vi "Calculate Friction Force.vi"(8 "error in":errorcluster, 10 "Mover Velocity in":refnum<class "PVector.lvclass">, 11 "Friction in":refnum<class "Friction.lvclass">) -> (0 "error out":errorcluster, 2 "Friction Force Out":refnum<class "PVector.lvclass">, 3 "Friction out":refnum<class "Friction.lvclass">)   [LabVIEW 2016, in "Friction.lvclass"]
uses:
  Friction.lvclass
  PVector/PVector.lvclass
  Friction.lvclass/Friction.ctl
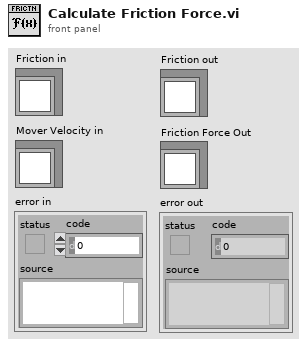
[diagram p1: front panel]
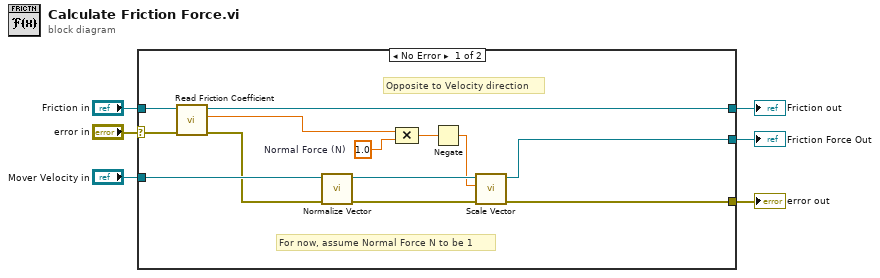
[diagram p0: block diagram]
diagram:
  n1 = case shown="No Error" "error in" {
    selector: "error in" -> [w17 w21]
    tunnel: [w9 w21] -> w5
    tunnel: [w18 w20] -> w3
    tunnel: "Friction in" -> [w19 w20]
    tunnel: [w10 _] -> w2
    tunnel: "Mover Velocity in" -> [w8 _]
    frame No Error {
      w13 = 1.0  # Normal Force (N)
      # "Opposite to Velocity direction"
      # "For now, assume Normal Force N to be 1"
      n2 = call "Read Friction Coefficient.vi"("error in"=w17, "Friction in"=w19) -> ("error out"=w7:errorcluster, "Friction Coefficient"=w14:dbl, "Friction out"=w18:refnum<class "Friction.lvclass">)  [unwired: 7 in]
      n3 = call "Normalize Vector.vi"("error in"=w7, "PVector in"=w8) -> ("error out"=w15:errorcluster, "norm(PVector) out"=w16:refnum<class "PVector.lvclass">)  [unwired: 8 in]
      n4 = Compound Arithmetic op=MULTIPLY(w14, w13) -> (w12:dbl)
      n5 = Negate(x=w12) -> (-x=w11:dbl)
      n6 = call "Scale Vector.vi"("error in"=w15, "n (1)"=w11, "PVector V"=w16) -> ("error out"=w9:errorcluster, "PVector nV"=w10:refnum<class "PVector.lvclass">)  [unwired: 7 in]
    }
    frame Error {
    }
  }
  "error out" <- w5
  "Friction out" <- w3
  "Friction Force Out" <- w2
